vi "公共界面++++++++++++++++.vi"(8 "错误输入（无错误）":errorcluster, 10 "界面切换队列":refnum<queue>, 11 "VISA资源名称输入":refnum<visa-resource-name>) -> (0 "错误输出":errorcluster, 3 "VISA资源名称输出":refnum<visa-resource-name>)   [LabVIEW 2018]
panel:
  out "毫秒计时值":u32
  in  "枚举":T1(ring)
  in  "选项卡控件":enum32{"选项卡 1", "选项卡 2"}(tab)
  out "DDT90356":dbl
  out "DDT90348":dbl
  out "自动界面":bool
  out "手动界面":bool
  out "参数界面":bool
  out "IO界面":bool
  out "产品界面":bool
  out "字符串":string
  out "DDT90352":dbl
  out "DDT90360":dbl
  out "通讯周期":dbl
  out "DT1184":T2(ring)
  # "X"
  # "Z1"
  # "Z2"
  # "Y"
  # "S"
  # "通讯周期"
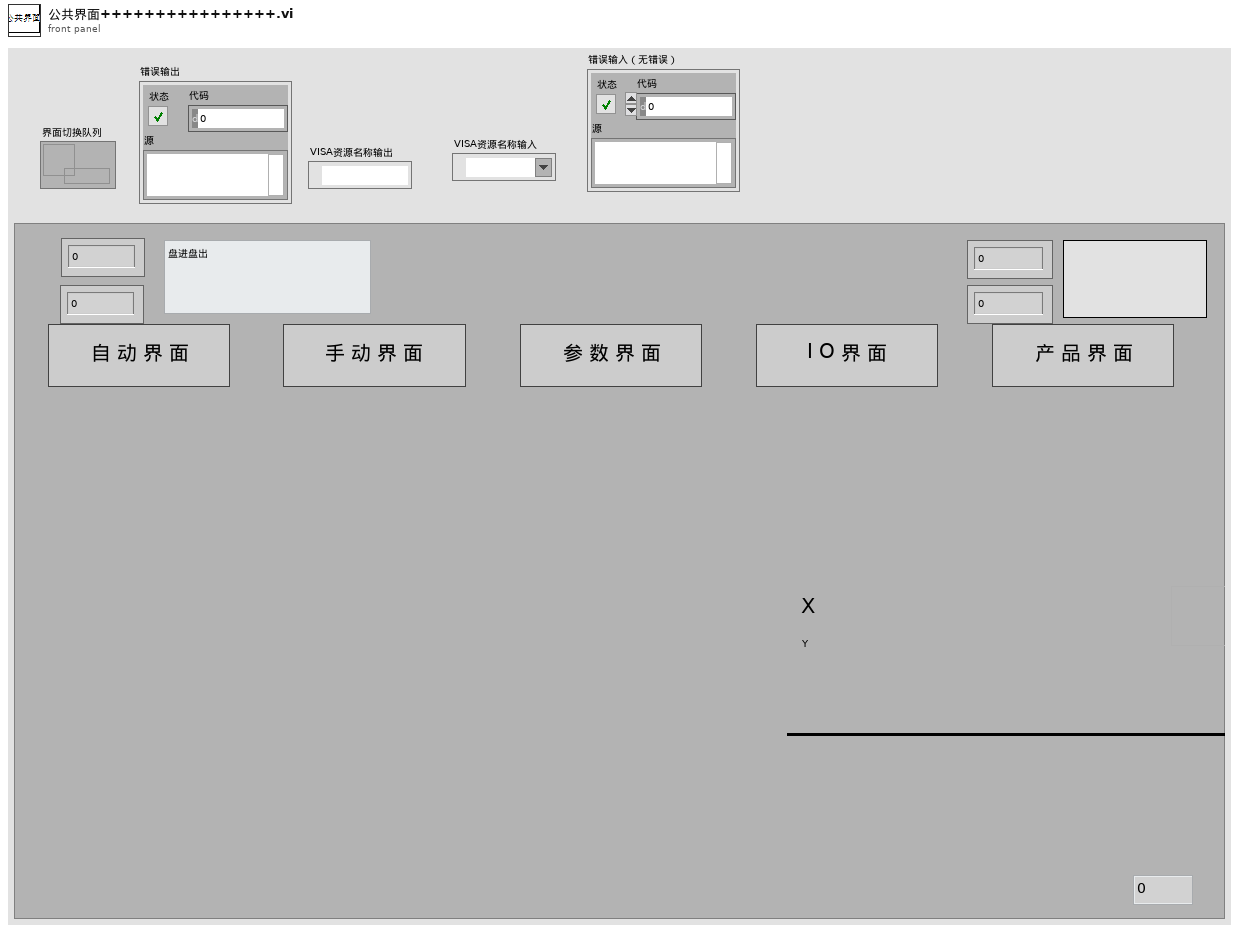
[diagram p1: front panel]
types:
  T1 = enum16{"读初始化", "读DDT90356", "读DT1184", "读DDT90348", ""}
  T2 = enum16{"盘进盘出", "卷进卷出", "盘进卷出", "管进盘出", "管进卷出", "卷进盘出", ""}
  T3 = enum8{"Enabled", "Disabled", "Disabled and Grayed Out"}
  T4 = typedef "数据簇.ctl" = cluster{"字符串":string, "数值":i32, "布尔":bool}
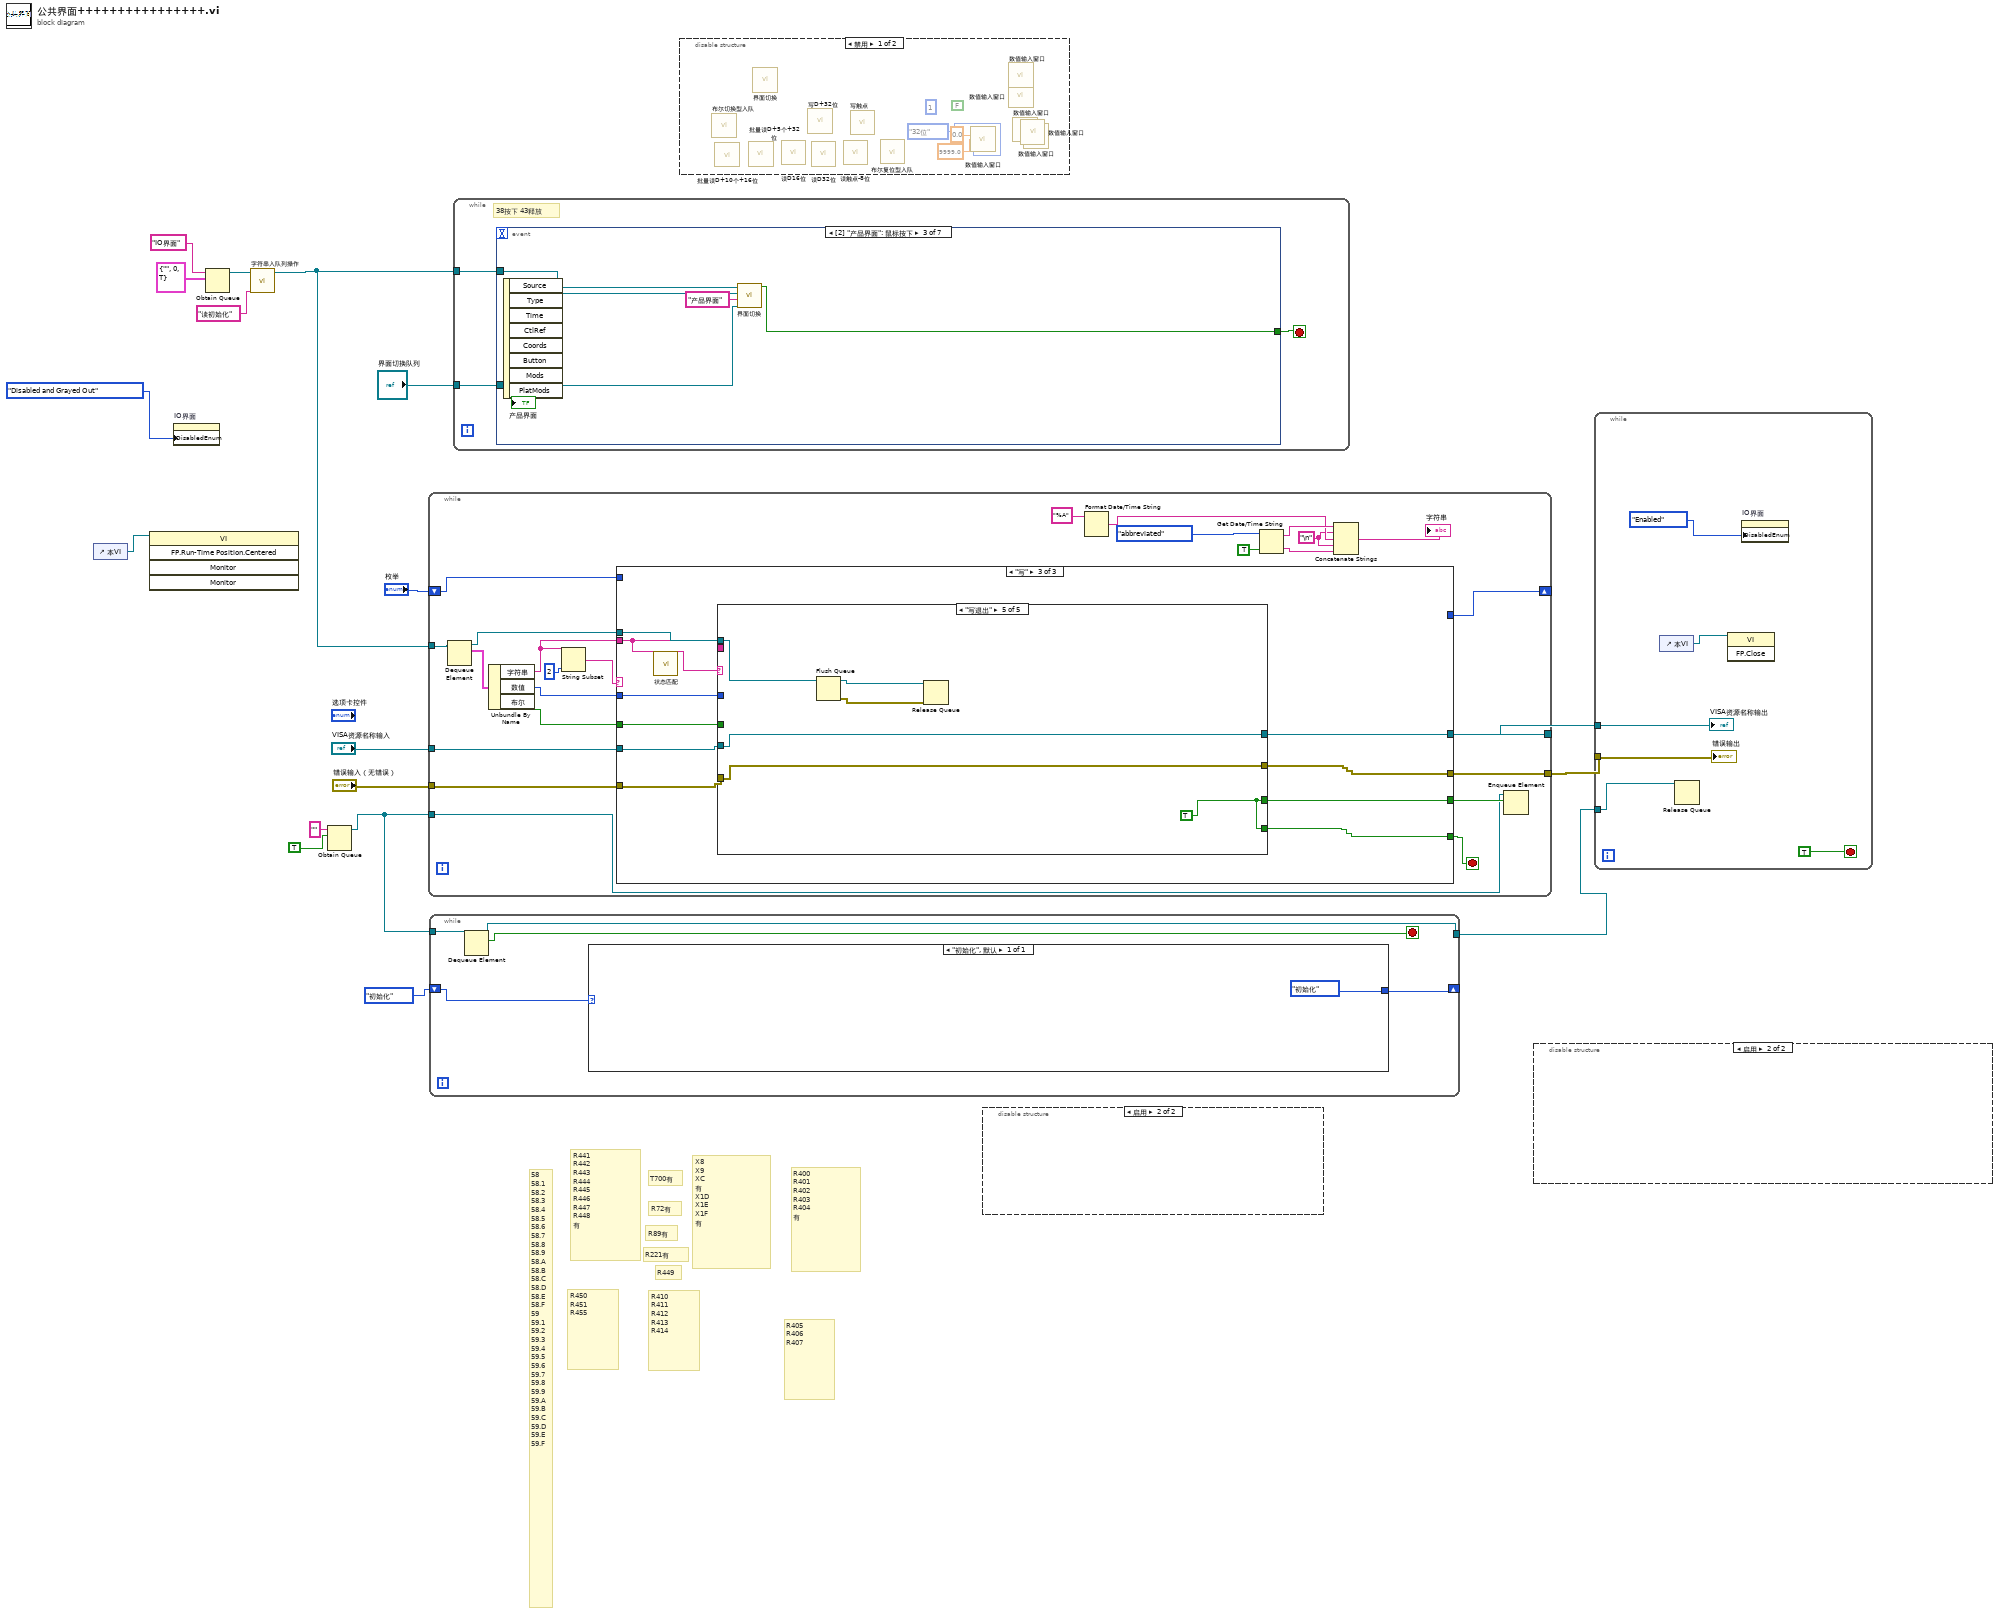
[diagram p0: block diagram]
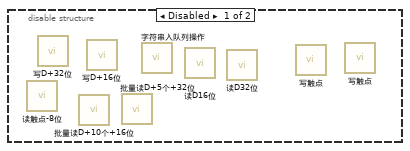
[diagram p19: hidden frame]
diagram:
  # "R449"
  # "R405\nR406\nR407"
  # "R410\nR411\nR412\nR413\nR414"
  # "R221有"
  # "R89有"
  # "R450\nR451\nR455"
  # "R72有"
  # "R441\nR442\nR443\nR444\nR445\nR446\nR447\nR448\n有"
  # "R400\nR401\nR402\nR403\nR404\n有"
  # "T700有"
  # "X8\nX9\nXC\n有\nX1D\nX1E\nX1F\n有"
  # "58\n58.1\n58.2\n58.3\n58.4\n58.5\n58.6\n58.7\n58.8\n58.9\n58.A\n58.B\n58.C\n58.D\n58.E\n58.F\n59\n59.1\n59.2\n59.3\n59.4\n59.5\n59.6\n59.7\n59.8\n59.9\n59.A\n59.B\n59.C\n59.D\n59.E\n59.F"
  n1 = control-ref of="本VI"() -> (w1:refnum<vi>)
  n2 = invoke class="VI" method="FP.Run-Time Position.Centered"(reference=w1) -> ()  [unwired: 4 in, 5 out]
  n3 = property on="IO界面" class="Bool"("DisabledEnum"=T3."Disabled and Grayed Out" ("禁用")) -> ()  [unwired: 2 in, 2 out]
  n4 = Obtain Queue(name (unnamed)="IO界面" ("名称（未命名）"), element data type=T4 {"字符串"="", "数值"=0, "布尔"=TRUE}) -> (queue out=w11:refnum<queue>)  [unwired: 3 in, 2 out]
  n5 = call "字符串入队列操作.vi"("字符消息入队列"="读初始化", "界面切换队列"=w11) -> ("队列输出"=w3:refnum<queue>)  [unwired: 9 in]
  n6 = Obtain Queue(name (unnamed)="" ("名称（未命名）"), element data type=TRUE) -> (queue out=w6:refnum<queue>)  [unwired: 3 in, 2 out]
  n7 = while {
    tunnel: w3 -> [w39]
    tunnel: "VISA资源名称输入" -> [w32]
    tunnel: "错误输入（无错误）" -> [w31]
    tunnel: [w30] -> w13
    tunnel: [w29] -> w12
    shift-right: [w26] -> _
    shift-left: "枚举" -> [w27]
    tunnel: w6 -> [w19]
    stop <- w21 stop-if-true
    w23 = "\n"
    n8 = Dequeue Element(queue=w39) -> (queue out=w36:refnum<queue>, element=w38:T4)  [unwired: 2 in, 2 out]
    n9 = Unbundle By Name(w38) -> ("字符串"=w33:string, "数值"=w35:i32, "布尔"=w34:bool)
    n10 = String Subset(string=w33, length (rest)=2 ("长度（剩余）")) -> (substring=w37:string)  [unwired: 1 in]
    n11 = case shown="\"写\"" w37 {
      selector: w37 -> [w46 _ _]
      tunnel: w36 -> [_ w54 w123]
      tunnel: w35 -> [_ w61 w122]
      tunnel: w34 -> [_ w60 w121]
      tunnel: w33 -> [_ _ w115]
      tunnel: w32 -> [w45 w59 w120]
      tunnel: w31 -> [w44 w58 w119]
      tunnel: [w45 w57 w117] -> w30
      tunnel: [w44 w56 w116] -> w29
      tunnel: [_ _ w118] -> w21
      tunnel: w27 -> [_ w52 _]
      tunnel: [_ w51 _] -> w26
      tunnel: [_ _ w113] -> w20
      frame "", Default {
        n12 = Concatenate Strings("无对应消息分支**" ("消息"), w46, "**" ("字符串"), "读写状态机" ("字符串")) -> (w48:string)
        n13 = One Button Dialog(message=w48) -> ()  [unwired: 1 in, 1 out]
      }
      frame "读" {
        n14 = case shown="\"读初始化\"" w52 {
          tunnel: w54 -> [_ _ _ _ _]
          tunnel: w61 -> [_ _ _ _ _]
          tunnel: w59 -> [w66 w78 w87 w100 w112]
          tunnel: w58 -> [w65 w77 w86 w99 w111]
          tunnel: [w66 w76 w85 w98 w112] -> w57
          tunnel: [w65 w75 w84 w97 w111] -> w56
          tunnel: w60 -> [_ _ _ _ _]
          tunnel: [_ _ _ _ TRUE] -> w53
          frame "读初始化" {
            n15 = Tick Count (ms)() -> (millisecond timer value=→"毫秒计时值":u32)
          }
          frame "读DDT90356" {
            n16 = call "批量读D+5个+32位.vi"("error out"=w77, "读取D地址"=90356, "VISA resource name out"=w78) -> ("error IO"=w75:errorcluster, "数组"=w81:i32[], "VISA resource name out 2"=w76:refnum<visa-resource-name>)  [unwired: 5 in, 1 out]
            n17 = Index Array(array=w81, index #1=0 ("索引"), index #2=2 ("索引")) -> (element #1=w74:i32, element #2=w73:i32)
            n18 = To Double Precision Float(number=w74) -> (double precision float=w72:dbl)
            n19 = To Double Precision Float(number=w73) -> (double precision float=w69:dbl)
            n20 = Divide(x=w72, y=100.0) -> (x/y=→"DDT90356":dbl)
            n21 = Divide(x=w69, y=100.0) -> (x/y=→"DDT90360":dbl)
          }
          frame "读DT1184" {
            n22 = call "读D16位.vi"("error out"=w86, "读取D地址"=1184, "VISA resource name out"=w87) -> ("error IO"=w84:errorcluster, "数值"=→"DT1184":u32, "VISA resource name out 2"=w85:refnum<visa-resource-name>)  [unwired: 5 in, 1 out]
          }
          frame "读DDT90348" {
            n23 = call "批量读D+5个+32位.vi"("error out"=w99, "读取D地址"=90348, "VISA resource name out"=w100) -> ("error IO"=w97:errorcluster, "数组"=w104:i32[], "VISA resource name out 2"=w98:refnum<visa-resource-name>)  [unwired: 5 in, 1 out]
            n24 = Index Array(array=w104, index #1=0 ("索引"), index #2=2 ("索引")) -> (element #1=w96:i32, element #2=w95:i32)
            n25 = To Double Precision Float(number=w95) -> (double precision float=w90:dbl)
            n26 = To Double Precision Float(number=w96) -> (double precision float=w94:dbl)
            n27 = Divide(x=w90, y=100.0) -> (x/y=→"DDT90352":dbl)
            n28 = Divide(x=w94, y=100.0) -> (x/y=→"DDT90348":dbl)
          }
          frame "" {
            n29 = local read "毫秒计时值"() -> (w108:u32)
            n30 = Tick Count (ms)() -> (millisecond timer value=w109:u32)
            n31 = Subtract(x=w109, y=w108) -> (x-y=w107:u32)
            n32 = Divide(x=w107, y=u32 1000) -> (x/y=→"通讯周期":dbl)
          }
        }
        n33 = case shown="假" w53 {
          tunnel: w52 -> [w63 _]
          tunnel: [w62 _] -> w51
          frame False {
            n34 = Increment(x=w63) -> (x+1=w62:T1)
          }
          frame True {
          }
        }
        n35 = call "字符串入队列操作.vi"("字符消息入队列"="读", "界面切换队列"=w54) -> ()  [unwired: 9 in, 1 out]
      }
      frame "写" {
        n36 = call "状态匹配.vi"("输入状态"=w115) -> ("输出状态"=w114:string)  [unwired: 10 in]
        n37 = case shown="\"写退出\"" w114 {
          selector: w114 -> [w126 _ _ _ _]
          tunnel: w123 -> [_ _ _ _ w166]
          tunnel: w122 -> [_ w132 w149 _ _]
          tunnel: w121 -> [_ _ _ w160 _]
          tunnel: w120 -> [w125 w142 w153 w165 w171]
          tunnel: w119 -> [w124 w141 w152 w164 w170]
          tunnel: [_ _ _ _ w169] -> w118
          tunnel: [w125 w140 w151 w163 w171] -> w117
          tunnel: [w124 w139 w150 w162 w170] -> w116
          tunnel: w115 -> [_ w131 w143 w154 _]
          tunnel: [_ _ _ _ w169] -> w113
          frame "", Default {
            n38 = Concatenate Strings("无对应消息分支**" ("消息"), w126, "**" ("字符串"), "写状态机" ("字符串")) -> (w130:string)
            n39 = One Button Dialog(message=w130) -> ()  [unwired: 1 in, 1 out]
          }
          frame "写DT" {
            n40 = String Length(string=w131) -> (length=w137:i32)
            n41 = Subtract(x=w137, y=4) -> (x-y=w135:i32)
            n42 = String Subset(string=w131, offset (0)=4 ("偏移量(0)"), length (rest)=w135) -> (substring=w134:string)
            n43 = Decimal String To Number(string=w134) -> (number=w133:i32)  [unwired: 2 in, 1 out]
            n44 = call "写D+16位.vi"("error out"=w141, "输入数值"=w132, "输入地址D"=w133, "VISA resource name out"=w142) -> ("error out 2"=w139:errorcluster, "VISA resource name out 2"=w140:refnum<visa-resource-name>)  [unwired: 3 in, 3 out]
          }
          frame "写DDT" {
            n45 = String Length(string=w143) -> (length=w147:i32)
            n46 = Subtract(x=w147, y=5) -> ()  [unwired: 1 out]
            n47 = String Subset(string=w143, offset (0)=5 ("偏移量(0)")) -> (substring=w144:string)  [unwired: 1 in]
            n48 = Decimal String To Number(string=w144) -> (number=w145:i32)  [unwired: 2 in, 1 out]
            n49 = call "写D+32位.vi"("error out"=w152, "输入数值"=w149, "输入地址D"=w145, "VISA resource name out"=w153) -> ("error out 2"=w150:errorcluster, "VISA resource name out 2"=w151:refnum<visa-resource-name>)  [unwired: 4 in, 2 out]
          }
          frame "写R" {
            n50 = String Length(string=w154) -> (length=w158:i32)
            n51 = Subtract(x=w158, y=3) -> (x-y=w156:i32)
            n52 = String Subset(string=w154, offset (0)=3 ("偏移量(0)"), length (rest)=w156) -> (substring=w155:string)
            n53 = call "写触点.vi"("布尔"=w160, "error out"=w164, "触点类型"="R", "写入起始地址"=w155, "VISA resource name out"=w165) -> ("error IO"=w162:errorcluster, "VISA resource name out 2"=w163:refnum<visa-resource-name>)  [unwired: 4 in, 1 out]
          }
          frame "写退出" {
            w169 = TRUE
            n54 = Flush Queue(queue=w166) -> (queue out=w167:refnum<queue>, error out=w168:errorcluster)  [unwired: 1 in, 1 out]
            n55 = Release Queue(queue=w167, error in (no error)=w168) -> ()  [unwired: 1 in, 3 out]
          }
        }
      }
    }
    n56 = Format Date/Time String(time format string (%c)="%A" ("时间格式字符串(%c)")) -> (date/time string=w24:string)  [unwired: 2 in]
    n57 = Get Date/Time String(date format (0)=enum16{"short", "long", "abbreviated"}."abbreviated" ("日期格式(0)"), want seconds? (F)=TRUE ("需要秒？(F)")) -> (date string=w41:string, time string=w22:string)  [unwired: 1 in]
    n58 = Concatenate Strings(w41, w23, w24, w23, w22) -> (→"字符串":string)
    n59 = Enqueue Element(queue=w19, element=w20) -> ()  [unwired: 2 in, 3 out]
  }
  n60 = while {
    shift-right: [w175] -> _
    shift-left: enum16{"初始化"}."初始化" -> [w176]
    tunnel: w6 -> [w174]
    tunnel: [w172] -> w5
    stop <- w173 stop-if-true
    n61 = Dequeue Element(queue=w174) -> (queue out=w172:refnum<queue>, element=w173:bool)  [unwired: 2 in, 2 out]
    n62 = case shown="\"初始化\", 默认" w176 {
      tunnel: [enum16{"初始化"}."初始化"] -> w175
      frame "初始化", Default {
      }
    }
  }
  n63 = while {
    tunnel: w3 -> [w179]
    tunnel: "界面切换队列" -> [w178]
    stop <- w180 stop-if-true
    # "38按下 43释放"
    n64 = event shown="[2] \"产品界面\": 鼠标按下" {
      selector: _ -> [_ _ _ _ _ _ _]
      dyn-events: _ -> [_ _ _ _ _ _ _]
      timeout: _ -> [_ _ _ _ _ _ _]
      tunnel: [w184 w186 w191 w196 w201 _ w208] -> w180
      tunnel: w179 -> [w185 w190 w195 w200 w205 _ w207]
      tunnel: w178 -> [w183 w189 w194 w199 w204 _ w206]
      event "IO界面": Mouse Down {
        n65 = event-data() -> ("CtlRef"=w182:refnum<vi>)  [unwired: 1 in, 7 out]
        n66 = call "界面切换.vi"("界面切换队列输入"=w183, "切换界面名称输入"="IO界面", "Bool引用句柄"=w182, "状态转移输入"=w185) -> ("布尔"=w184:bool)  [unwired: 7 in]
      }
      event "参数界面": Mouse Down {
        n67 = event-data() -> ("CtlRef"=w188:refnum<vi>)  [unwired: 1 in, 7 out]
        n68 = call "界面切换.vi"("界面切换队列输入"=w189, "切换界面名称输入"="参数界面", "Bool引用句柄"=w188, "状态转移输入"=w190) -> ("布尔"=w186:bool)  [unwired: 7 in]
      }
      event "产品界面": Mouse Down {
        n69 = event-data() -> ("CtlRef"=w193:refnum<vi>)  [unwired: 1 in, 7 out]
        n70 = call "界面切换.vi"("界面切换队列输入"=w194, "切换界面名称输入"="产品界面", "Bool引用句柄"=w193, "状态转移输入"=w195) -> ("布尔"=w191:bool)  [unwired: 7 in]
      }
      event "手动界面": Mouse Down {
        n71 = event-data() -> ("CtlRef"=w198:refnum<vi>)  [unwired: 1 in, 7 out]
        n72 = call "界面切换.vi"("界面切换队列输入"=w199, "切换界面名称输入"="手动界面", "Bool引用句柄"=w198, "状态转移输入"=w200) -> ("布尔"=w196:bool)  [unwired: 7 in]
      }
      event "自动界面": Mouse Down {
        n73 = event-data() -> ("CtlRef"=w203:refnum<vi>)  [unwired: 1 in, 7 out]
        n74 = call "界面切换.vi"("界面切换队列输入"=w204, "切换界面名称输入"="自动界面", "Bool引用句柄"=w203, "状态转移输入"=w205) -> ("布尔"=w201:bool)  [unwired: 7 in]
      }
      event Timeout {
        n75 = event-data() -> ()  [unwired: 1 in, 3 out]
      }
      event Panel Close? {
        n76 = event-data() -> ()  [unwired: 1 in, 4 out]
        n77 = Two Button Dialog(message="确定退出程序？" ("消息")) -> (T button?=w209:bool)  [unwired: 2 in]
        n78 = case shown="真" w209 {
          tunnel: [_ TRUE] -> w208
          tunnel: w207 -> [_ w214]
          tunnel: w206 -> [_ w213]
          frame False {
          }
          frame True {
            n79 = call "字符串入队列操作.vi"("字符消息入队列"="退出", "界面切换队列"=w213) -> ()  [unwired: 9 in, 1 out]
            n80 = call "字符串入队列操作.vi"("字符消息入队列"="写退出", "界面切换队列"=w214) -> ()  [unwired: 9 in, 1 out]
          }
        }
        n81 = event-data("Discard?"=TRUE ("放弃？")) -> ()  [unwired: 1 in, 1 out]
      }
    }
  }
  n82 = disable-structure shown="禁用" {
    frame Disabled {
      (unwired) u32 1 ("转换比例")
      (unwired) FALSE ("忽略数值上下限")
      n83 = call "布尔切换型入队.vi"() -> ()  [unwired: 12 in]
      n84 = call "批量读D+10个+16位.vi"() -> ()  [unwired: 8 in, 4 out]
      n85 = call "批量读D+5个+32位.vi"() -> ()  [unwired: 8 in, 4 out]
      n86 = call "界面切换.vi"() -> ()  [unwired: 11 in, 1 out]
      n87 = call "读D16位.vi"() -> ()  [unwired: 8 in, 4 out]
      n88 = call "写D+32位.vi"() -> ()  [unwired: 8 in, 4 out]
      n89 = call "读D32位.vi"() -> ()  [unwired: 9 in, 3 out]
      n90 = call "读触点-8位.vi"() -> ()  [unwired: 8 in, 4 out]
      n91 = call "写触点.vi"() -> ()  [unwired: 9 in, 3 out]
      n92 = call "布尔复位型入队.vi"() -> ()  [unwired: 6 in, 3 out]
      n93 = call "数值输入窗口.vi"("输入下限"=0.0, "输入上限"=9999.0, "数据类型"=enum16{"32位", "16位"}."32位") -> ("转换比例"=w220:u32)  [unwired: 9 in, 3 out]
      n94 = call "数值输入窗口.vi"() -> ()  [unwired: 13 in, 3 out]
      n95 = call "数值输入窗口.vi"() -> ()  [unwired: 13 in, 3 out]
      n96 = call "数值输入窗口.vi"() -> ()  [unwired: 13 in, 3 out]
      n97 = call "数值输入窗口.vi"() -> ()  [unwired: 13 in, 3 out]
      n98 = call "数值输入窗口.vi"() -> ()  [unwired: 13 in, 3 out]
    }
    frame Enabled {
    }
  }
  n99 = disable-structure shown="启用" {
    frame Disabled {
      n100 = call "读触点-8位.vi"() -> ()  [unwired: 8 in, 4 out]
      n101 = call "写D+32位.vi"() -> ()  [unwired: 8 in, 4 out]
      n102 = call "批量读D+10个+16位.vi"() -> ()  [unwired: 8 in, 4 out]
      n103 = call "写D+16位.vi"() -> ()  [unwired: 7 in, 5 out]
      n104 = call "批量读D+5个+32位.vi"() -> ()  [unwired: 8 in, 4 out]
      n105 = call "字符串入队列操作.vi"() -> ()  [unwired: 11 in, 1 out]
      n106 = call "读D16位.vi"() -> ()  [unwired: 8 in, 4 out]
      n107 = call "读D32位.vi"() -> ()  [unwired: 9 in, 3 out]
      n108 = call "写触点.vi"() -> ()  [unwired: 9 in, 3 out]
      n109 = call "写触点.vi"() -> ()  [unwired: 9 in, 3 out]
    }
    frame Enabled {
    }
  }
  n110 = disable-structure shown="启用" {
    frame Disabled {
      n111 = for {
        i -> [w222]
        n112 = case shown="9" w222 {
          frame 0, Default {
          }
          frame 1 {
          }
          frame 2 {
          }
          frame 3 {
          }
          frame 4 {
          }
          frame 5 {
          }
          frame 6 {
          }
          frame 7 {
          }
          frame 8 {
          }
          frame 9 {
          }
        }
      }
      n113 = for {
        i -> [w221]
        n114 = case shown="7" w221 {
          frame 0, Default {
          }
          frame 1 {
          }
          frame 2 {
          }
          frame 3 {
          }
          frame 4 {
          }
          frame 5 {
          }
          frame 6 {
          }
          frame 7 {
          }
        }
      }
    }
    frame Enabled {
    }
  }
  n115 = while {
    tunnel: w13 -> [w226]
    tunnel: w12 -> [w225]
    tunnel: w5 -> [w224]
    stop <- TRUE stop-if-true
    n116 = control-ref of="本VI"() -> (w227:refnum<vi>)
    n117 = Release Queue(queue=w224) -> ()  [unwired: 2 in, 3 out]
    n118 = invoke class="VI" method="FP.Close"(reference=w227) -> ()  [unwired: 2 in, 3 out]
    n119 = property on="IO界面" class="Bool"("DisabledEnum"=T3."Enabled" ("禁用")) -> ()  [unwired: 2 in, 2 out]
    "VISA资源名称输出" <- w226
    "错误输出" <- w225
  }
